vi "controlRoomLoop.vi"() -> ()   [LabVIEW 2018]
uses:
  <vilib>/Platform/TimedLoop/XDataNode/timing_clust.ctl
  <vilib>/Platform/TimedLoop/XDataNode/nitl_modes.ctl
  <vilib>/Platform/TimedLoop/XDataNode/wakeup.ctl
  <vilib>/platform/TimedLoop/XDataNode/XDataNode.xnode
  <vilib>/Platform/TimedLoop/XDataNode/XDNodeRunTimeDep.lvlib
panel:
  in  "Climb Stilt Period":i64=50
  in  "SensorsPeriod":i64=50
  in  "limelightPeriod":i64=50
  in  "HatchPannelPeriod":i64=100
  in  "Drive Period":i64=20
  in  "ClimbPeriod":i64=50
  in  "CargoPeriod":i64=30
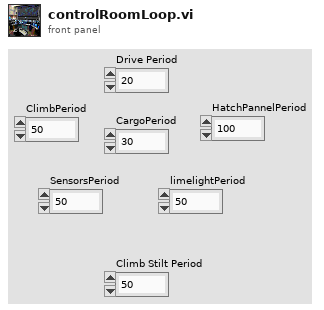
[diagram p1: front panel]
types:
  T1 = typedef "XDNodeRunTimeDep.lvlib/timing_clust.ctl" = cluster{"Expected End [f-1]":u64, "Actual End [f-1]":u64, "Finished Late? [f-1]":bool, "Expected End [i-1]":u64, "Actual End [i-1]":u64, "Finished Late? [i-1]":bool, "Expected Start [i]":u64, "Actual Start [i]":u64, "Expected Start [f]":u64, "Actual Start [f]":u64, "Source Name":string, "Structure Name":string, "Period":i64, "Deadline":i64, "Offset":i64, "Start":i64, "Priority":i32, "Timeout":i32, "Mode":T2, "Wakeup Reason":T3, "Error":errorcluster, "Source Type":string, "Secondary Source Type":string, "Global End Time":u64, "Global Start Time":u64, "Frame Duration":u64, "Iteration Duration":u64, "Assigned CPU":i32, "I/O Scan Engine Mode":u32}
  T2 = typedef "XDNodeRunTimeDep.lvlib/nitl_modes.ctl" = enum32{"No Change", "Process missed periods, maintain original phase", "Discard missed periods, maintain original phase", "Process missed periods, ignore original phase", "Discard missed periods, ignore original phase"}
  T3 = typedef "XDNodeRunTimeDep.lvlib/wakeup.ctl" = enum32{"Normal", "Aborted", "Asynchronous wakeup", "Timing source error", "Timed loop error", "Timeout"}
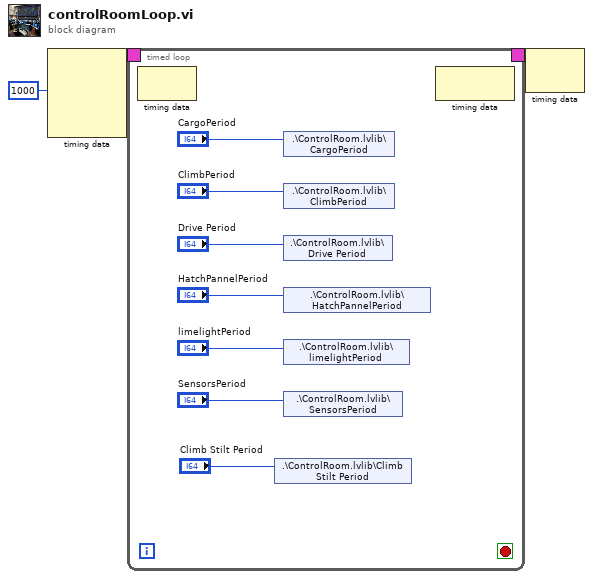
[diagram p0: block diagram]
diagram:
  n1 = node-c288(i64 1000 ("Period")) -> (w3:T1)  [unwired: 3 in]
  n2 = timed-loop {
    timing: w3 -> [_]
    timing-out: [_] -> w2
    stop <- _ stop-if-true
    n3 = node-c288() -> ()  [unwired: 1 in, 1 out]
    n4 = shared-variable ".\\ControlRoom.lvlib\\Climb Stilt Period"("Climb Stilt Period") -> ()  [unwired: 1 in, 1 out]
    n5 = shared-variable ".\\ControlRoom.lvlib\\CargoPeriod"("CargoPeriod") -> ()  [unwired: 1 in, 1 out]
    n6 = shared-variable ".\\ControlRoom.lvlib\\ClimbPeriod"("ClimbPeriod") -> ()  [unwired: 1 in, 1 out]
    n7 = shared-variable ".\\ControlRoom.lvlib\\Drive Period"("Drive Period") -> ()  [unwired: 1 in, 1 out]
    n8 = shared-variable ".\\ControlRoom.lvlib\\HatchPannelPeriod"("HatchPannelPeriod") -> ()  [unwired: 1 in, 1 out]
    n9 = shared-variable ".\\ControlRoom.lvlib\\limelightPeriod"("limelightPeriod") -> ()  [unwired: 1 in, 1 out]
    n10 = shared-variable ".\\ControlRoom.lvlib\\SensorsPeriod"("SensorsPeriod") -> ()  [unwired: 1 in, 1 out]
    n11 = node-c288() -> ()  [unwired: 1 in, 1 out]
  }
  n12 = node-c288(w2) -> ()  [unwired: 1 out]
